vi "Set Magnet Vector.vi"(8 "error in (no error)":errorcluster, 9 "Target Rate Limit (T/min)":dbl, 10 "Target Field (T)":dbl[](array[numeric]), 11 "Instrument.VRM in":refnum<class "Instrument.OxfordVRM.lvclass">) -> (0 "error out":errorcluster, 3 "Instrument.VRM out":refnum<class "Instrument.OxfordVRM.lvclass">)   [LabVIEW 2019, in "Instrument.OxfordVRM.lvclass"]
uses:
  Instrument.OxfordVRM.lvclass
  C:/Program Files (x86)/National Instruments/LabVIEW 2019/user.lib/LevyLab/Instrument Framework/Instrument/Instrument.lvclass
  Set Vector Magnet.vi/5e873d59-b7fa-4b76-b36a-7150f831c1b5.vi/149fcd9c-dedd-4ff1-9a94-39a9576e844c.vi
  Set Vector Magnet.vi/5e873d59-b7fa-4b76-b36a-7150f831c1b5.vi/149fcd9c-dedd-4ff1-9a94-39a9576e844c.vi/069cb1ff-1a2e-4715-878d-17cae921945f.vi
  Set Vector Magnet.vi/5e873d59-b7fa-4b76-b36a-7150f831c1b5.vi/149fcd9c-dedd-4ff1-9a94-39a9576e844c.vi/9a24557b-199f-4ef9-9934-e7afc38a5181.vi
  <userlib>/LevyLab/Instrument Framework/Instrument/API/Remote Client.vi
  <vilib>/Utility/Data Type/Get Type Information.vi
  <vilib>/JDP Science/JSONtext/JSON text to Variant.vi
  <vilib>/JDP Science/JSONtext/LVClass Serializer/JSONtext LVClass Serializer.lvclass
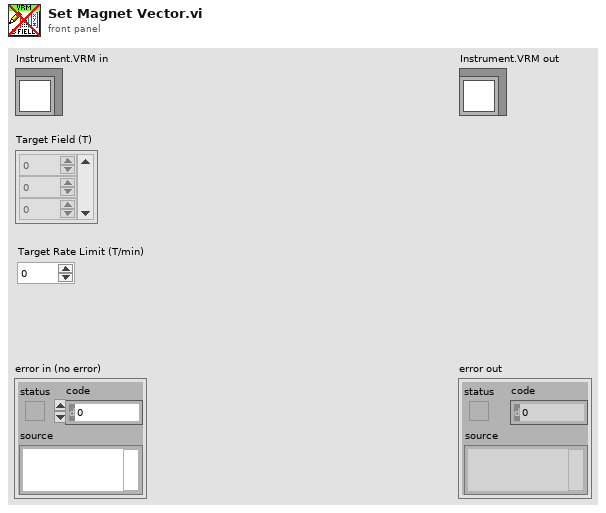
[diagram p1: front panel]
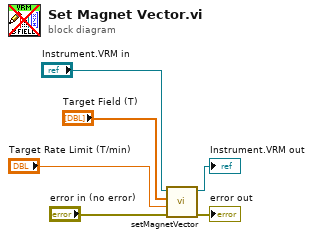
[diagram p0: block diagram]
diagram:
  n1 = call-dynamic "setMagnetVector.vi"("error in (no error)"="error in (no error)", "Target Rate Limit (T/min)"="Target Rate Limit (T/min)", "Target Field (T)"="Target Field (T)", "Instrument.VRM in"="Instrument.VRM in") -> ("error out"=→"error out":errorcluster, "Instrument.VRM out"=→"Instrument.VRM out":refnum<class "Instrument.OxfordVRM.lvclass">)  [unwired: 6 in]
